vi "Write No. of steps.vi"(8 "error in (no error)":errorcluster, 10 "No. of steps":u32, 11 "Scan SBlock in":refnum<class "Scan SBlock.lvclass">) -> (0 "error out":errorcluster, 3 "Scan SBlock out":refnum<class "Scan SBlock.lvclass">)   [LabVIEW 2020, in "Run Utilities.lvlib" / "Scan SBlock.lvclass"]
uses:
  Scan SBlock.lvclass
  Scan SBlock.lvclass/Scan SBlock.ctl
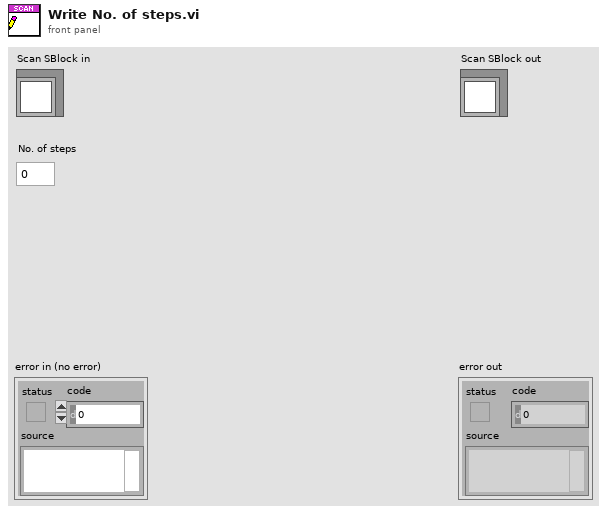
[diagram p1: front panel]
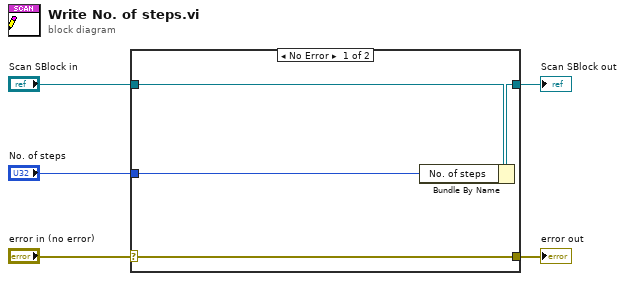
[diagram p0: block diagram]
diagram:
  n1 = case shown="No Error" "error in (no error)" {
    selector: "error in (no error)" -> [w9 w10]
    tunnel: [w9 w10] -> w4
    tunnel: [w7 w11] -> w2
    tunnel: "Scan SBlock in" -> [w8 w11]
    tunnel: "No. of steps" -> [w6 _]
    frame No Error {
      n2 = Bundle By Name(cluster=w8, "No. of steps"=w6) -> (w7:refnum<class "Scan SBlock.lvclass">)
    }
    frame Error {
    }
  }
  "error out" <- w4
  "Scan SBlock out" <- w2
